vi "UpdatePlotData.vi"(8 "DataArrayIn":dbl[][](array[numeric])=[[0.0, 0.0], [0.0, 0.0], [1.0, 2.0], [0.0, 0.0]], 9 "TimeArrayIn":dbl[](array[numeric])=[0.0, 0.0], 10 "DataReturn":string[](array[string])=["1", "2", "3", "4", "5"], 11 "PlotCount":i32=2) -> (0 "DataArrayOut":dbl[][](array[numeric])=[[0.0, 1.0], [0.0, 2.0], [2.0, 3.0], [0.0, 4.0]], 1 "TimeArrayOut":dbl[](array[numeric]))   [LabVIEW 2012]
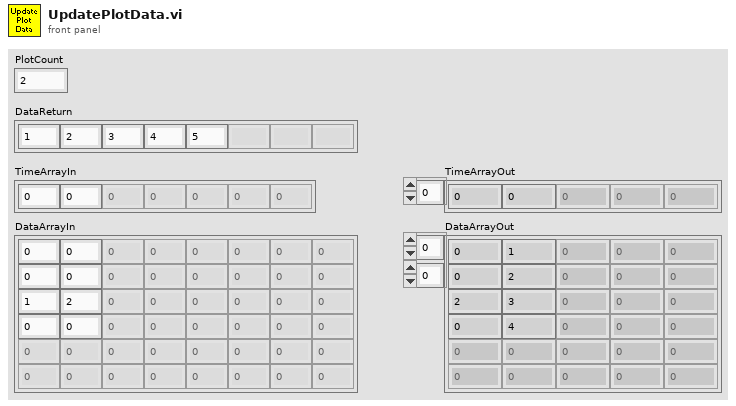
[diagram p1: front panel]
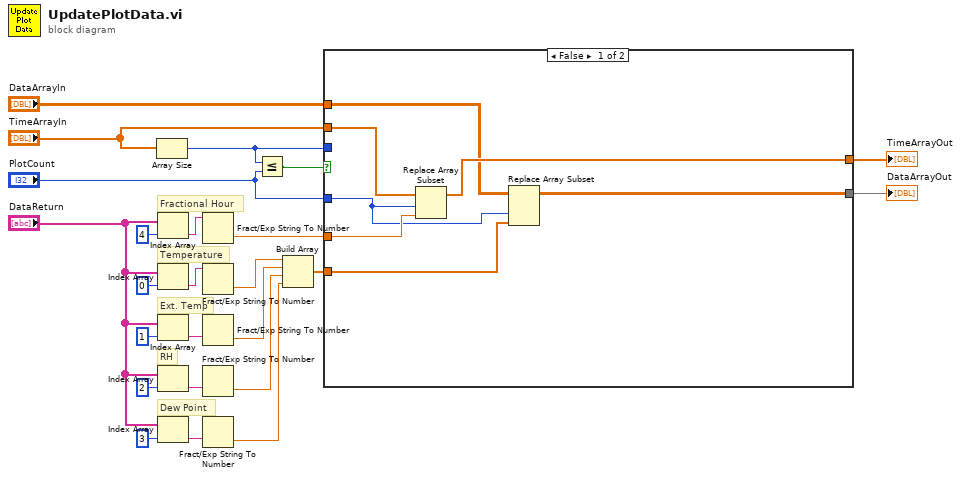
[diagram p0: block diagram]
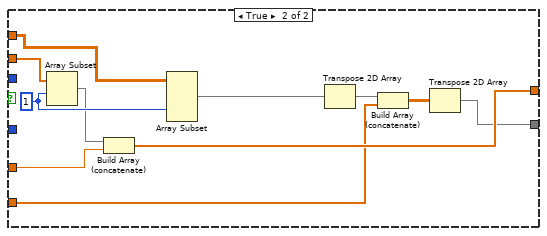
[diagram p2: hidden frame]
diagram:
  # "Dew Point"
  # "RH"
  # "Ext. Temp"
  # "Temperature"
  # "Fractional Hour"
  n1 = Array Size(array="TimeArrayIn") -> (size(s)=w11:i32)
  n2 = Index Array(array="DataReturn", index=4) -> (element=w23:string)
  n3 = Index Array(array="DataReturn", index=0) -> (element=w16:string)
  n4 = Index Array(array="DataReturn", index=1) -> (element=w14:string)
  n5 = Index Array(array="DataReturn", index=2) -> (element=w9:string)
  n6 = Index Array(array="DataReturn", index=3) -> (element=w7:string)
  n7 = Fract/Exp String To Number(string=w23) -> (number=w19:dbl)  [unwired: 3 in, 1 out]
  n8 = Fract/Exp String To Number(string=w16) -> (number=w5:dbl)  [unwired: 3 in, 1 out]
  n9 = Fract/Exp String To Number(string=w14) -> (number=w4:dbl)  [unwired: 3 in, 1 out]
  n10 = Fract/Exp String To Number(string=w9) -> (number=w3:dbl)  [unwired: 3 in, 1 out]
  n11 = Fract/Exp String To Number(string=w7) -> (number=w2:dbl)  [unwired: 3 in, 1 out]
  n12 = Less Or Equal?(x=w11, y="PlotCount") -> (x <= y?=w22:bool)
  n13 = Build Array(w5, w4, w3, w2) -> (w1:dbl[])
  n14 = case shown="False" w22 {
    tunnel: "TimeArrayIn" -> [w31 w42]
    tunnel: "PlotCount" -> [w27 _]
    tunnel: w19 -> [w30 w39]
    tunnel: "DataArrayIn" -> [w28 w37]
    tunnel: [w26 w35] -> w13
    tunnel: [w29 w38] -> w12
    tunnel: w11 -> [_ _]
    tunnel: w1 -> [w25 w32]
    frame False {
      n15 = Replace Array Subset(array=w31, new element=w30, index=w27) -> (w29:dbl[])
      n16 = Replace Array Subset(array=w28, new element=w25, index (col)=w27) -> (w26:dbl[][])  [unwired: 1 in]
    }
    frame True {
      w41 = 1 ("length")
      n17 = Array Subset(array=w42, index=w41) -> (w40:dbl[])  [unwired: 1 in]
      n18 = Build Array (concatenate)(w40, w39) -> (w38:dbl[])
      n19 = Array Subset(array=w37, index (col)=w41) -> (w34:dbl[][])  [unwired: 3 in]
      n20 = Transpose 2D Array(2D array=w34) -> (transposed array=w33:dbl[][])
      n21 = Build Array (concatenate)(w33, w32) -> (w36:dbl[][])
      n22 = Transpose 2D Array(2D array=w36) -> (transposed array=w35:dbl[][])
    }
  }
  "DataArrayOut" <- w13
  "TimeArrayOut" <- w12
